vi "getPhysicalChannels.vi"(8 "error in (no error)":errorcluster, 11 "DigitalOutput.lvclass in":refnum<class "DigitalOutput.lvclass">) -> (0 "error out":errorcluster, 2 "Physical Channels":string, 3 "DigitalOutput.lvclass out":refnum<class "DigitalOutput.lvclass">)   [LabVIEW 2009, in "Hardware.lvlib" / "Channels.lvlib" / "DigitalOutput.lvclass"]
uses:
  DigitalOutput.lvclass
  DigitalOutput.lvclass/DigitalOutput.ctl
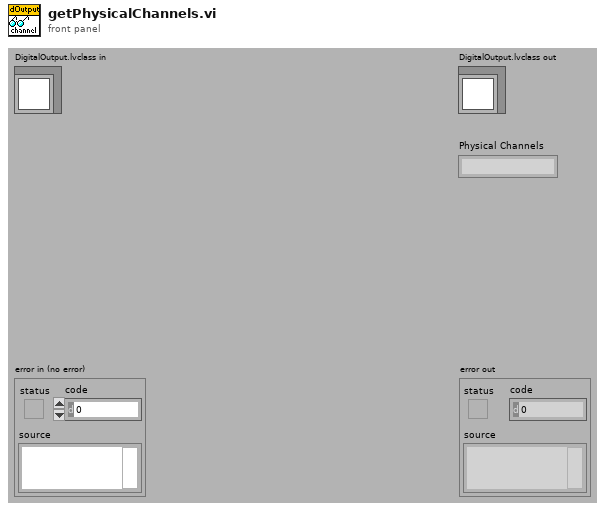
[diagram p1: front panel]
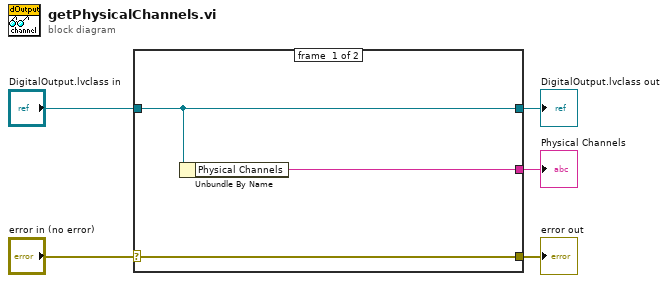
[diagram p0: block diagram]
diagram:
  n1 = case shown="No Error" "error in (no error)" {
    selector: "error in (no error)" -> [w8 w9]
    tunnel: [w8 w9] -> w4
    tunnel: [w7 w10] -> w2
    tunnel: "DigitalOutput.lvclass in" -> [w7 w10]
    tunnel: [w6 _] -> w1
    frame #0 {
      n2 = Unbundle By Name(w7) -> ("Physical Channels"=w6:string)
    }
    frame #1 {
    }
  }
  "error out" <- w4
  "DigitalOutput.lvclass out" <- w2
  "Physical Channels" <- w1
